vi "read_relay_card.vi"(1 "Slot":i32=10 min=0 max=14) -> (0 "data":string)   [LabVIEW 2011]
uses:
  globals.vi
panel:
  out "error out 2":errorcluster
  out "error out":errorcluster
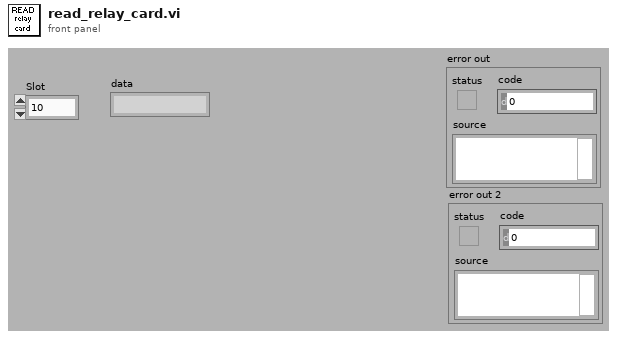
[diagram p1: front panel]
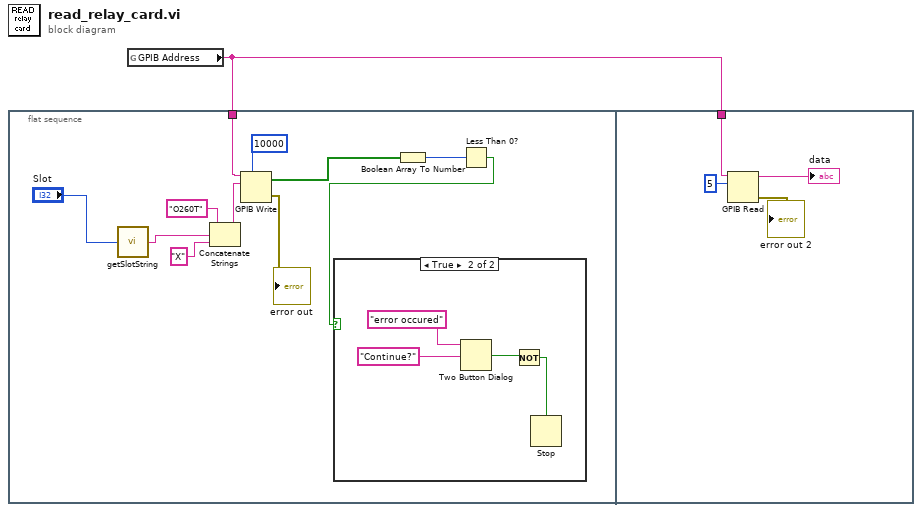
[diagram p0: block diagram]
diagram:
  n1 = flat-sequence {
    tunnel: w1 -> [w9]
    tunnel: w1 -> [w19]
    frame #0 {
      n2 = call "getSlotString.vi"("Slot"="Slot") -> ("string"=w2:string)
      n3 = Concatenate Strings("O260T" ("string"), w2, "X" ("string")) -> (w12:string)
      n4 = GPIB Write(0:w9, 1:w12, 4:10000 ("timeout ms (488.2 global)")) -> (5:w7:bool[], 6:→"error out":errorcluster)  [unwired: 1 in, 1 out]
      n5 = Boolean Array To Number(Boolean array=w7) -> (number=w6:u32)
      n6 = Less Than 0?(x=w6) -> (x < 0?=w5:bool)
      n7 = case shown="True" w5 {
        frame False {
        }
        frame True {
          n8 = Two Button Dialog(message="error occured", 2:"Continue?" ("T button name (\"OK\")")) -> (T button?=w14:bool)  [unwired: 1 in]
          n9 = Not(x=w14) -> (.not. x?=w13:bool)
          n10 = Stop(stop? (T)=w13) -> ()
        }
      }
    }
    frame #1 {
      n11 = GPIB Read(0:w19, 1:5 ("byte count")) -> (5:→"data":string, 7:→"error out 2":errorcluster)  [unwired: 1 in, 3 out]
    }
  }
  n12 = global read "globals.vi" "GPIB Address"() -> (w1:string)
